vi "总磷总氮量程读取.vi"(8 "error in (no error)":errorcluster caption="错误输入（无错误）", 11 "测量参数":u16(ring) items=["COD"=22, "氨氮"=3, "总氮"=2, "总磷"=1]) -> (0 "error out":errorcluster caption="错误输出", 3 "量程参数读取":T1)   [LabVIEW 2016, in "斯坦道通用流路CODmn.lvlib"]
panel:
  out "第二个子数组":u16[](array[numeric]) format="%4x"
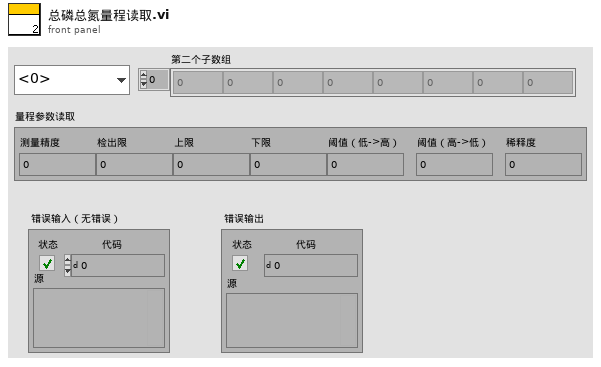
[diagram p1: front panel]
types:
  T1 = cluster{"测量精度":u16, "检出限":dbl, "上限":dbl, "下限":dbl, "阈值（低->高）":dbl, "阈值（高->低）":dbl, "稀释度":dbl}
  T2 = cluster{"FLOAT[0]":sgl, "FLOAT[1]":sgl, "FLOAT[2]":sgl, "FLOAT[3]":sgl, "FLOAT[4]":sgl}
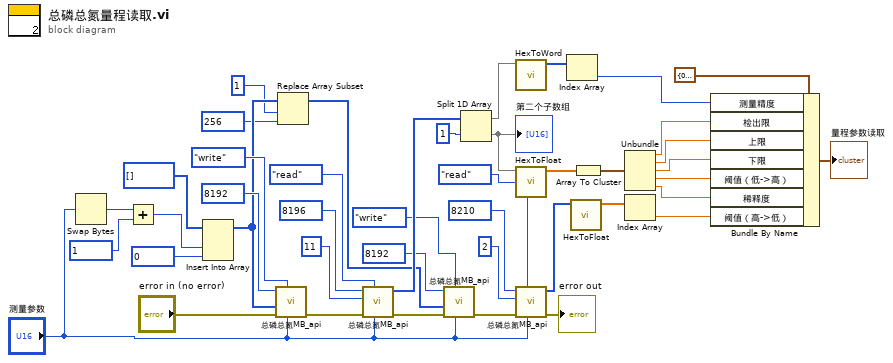
[diagram p0: block diagram]
diagram:
  n1 = Swap Bytes(anything="测量参数") -> (byte swapped=w1:u16)
  n2 = Add(x=w1, y=u16 1 ("starting address")) -> (x+y=w39:u16)
  n3 = Insert Into Array(array=u16[] [] ("数组"), new element #1=w39, new element #2=u16 0 ("starting address")) -> (w12:u16[])  [unwired: 1 in]
  n4 = call "总磷总氮MB_api.vi"("Slave ID"="测量参数", "STEP"=enum16{"open", "read", "write", "close"}."write", "Error in"="error in (no error)", "values"=w12, "starting address"=u16 8192) -> ("error out"=w35:errorcluster)  [unwired: 4 in, 2 out]
  n5 = Replace Array Subset(array=w12, new element=u16 256 ("starting address"), index=1 ("索引")) -> (w10:u16[])
  n6 = call "总磷总氮MB_api.vi"("Slave ID"="测量参数", "STEP"=enum16{"open", "read", "write", "close"}."read", "Error in"=w35, "quantity"=u16 11, "starting address"=u16 8196) -> ("error out"=w22:errorcluster, "Registers"=w32:u16[])  [unwired: 4 in, 1 out]
  n7 = call "总磷总氮MB_api.vi"("Slave ID"="测量参数", "STEP"=enum16{"open", "read", "write", "close"}."write", "Error in"=w22, "values"=w10, "starting address"=u16 8192) -> ("error out"=w21:errorcluster)  [unwired: 4 in, 2 out]
  n8 = Split 1D Array(array=w32, index=1 ("长度")) -> (first subarray=w9:u16[], second subarray=w8:u16[])
  "第二个子数组" <- w8
  n9 = call "HexToWord.vi"("数组"=w9) -> ("WORD"=w30:u16[])  [unwired: 10 in]
  n10 = call "HexToFloat.vi"("数组"=w8) -> ("FLOAT"=w42:sgl[])  [unwired: 10 in]
  n11 = call "总磷总氮MB_api.vi"("Slave ID"="测量参数", "STEP"=enum16{"open", "read", "write", "close"}."read", "Error in"=w21, "quantity"=u16 2, "starting address"=u16 8210) -> ("error out"=→"error out":errorcluster, "Registers"=w14:u16[])  [unwired: 4 in, 1 out]
  n12 = Index Array(array=w30) -> (element=w29:u16)  [unwired: 1 in]
  n13 = call "HexToFloat.vi"("数组"=w14) -> ("FLOAT"=w13:sgl[])  [unwired: 10 in]
  n14 = Array To Cluster(array=w42) -> (cluster=w28:T2)
  n15 = Unbundle(w28) -> ("FLOAT[0]"=w27:sgl, "FLOAT[1]"=w26:sgl, "FLOAT[2]"=w25:sgl, "FLOAT[3]"=w24:sgl, "FLOAT[4]"=w23:sgl)
  n16 = Index Array(array=w13) -> (element=w5:sgl)  [unwired: 1 in]
  n17 = Bundle By Name(cluster=T1 {"测量精度"=0, "检出限"=0.0, "上限"=0.0, "下限"=0.0, "阈值（低->高）"=0.0, "阈值（高->低）"=0.0, "稀释度"=0.0} ("量程参数读取"), "测量精度"=w29, "检出限"=w27, "上限"=w26, "下限"=w25, "阈值（低->高）"=w24, "稀释度"=w23, "阈值（高->低）"=w5) -> (→"量程参数读取":T1)
